vi "Substract Background.vi"(4 "Background":T1, 5 "Substract":u16(ring) items=["None", "Background", "Reference"], 6 "error in (no error)":errorcluster, 7 "Reference":T1, 8 "Dest Img":T1, 9 "Region of Interest":i32[](array[numeric])=[-1, -1, 32000, 32000], 10 "Image Src":T1) -> (0 "error out":errorcluster, 3 "Img Out":T1)   [LabVIEW 2013]
uses:
  <vilib>/vision/Image Controls.llb/IMAQ Image.ctl
  <vilib>/vision/NI_Vision_Development_Module.lvlib
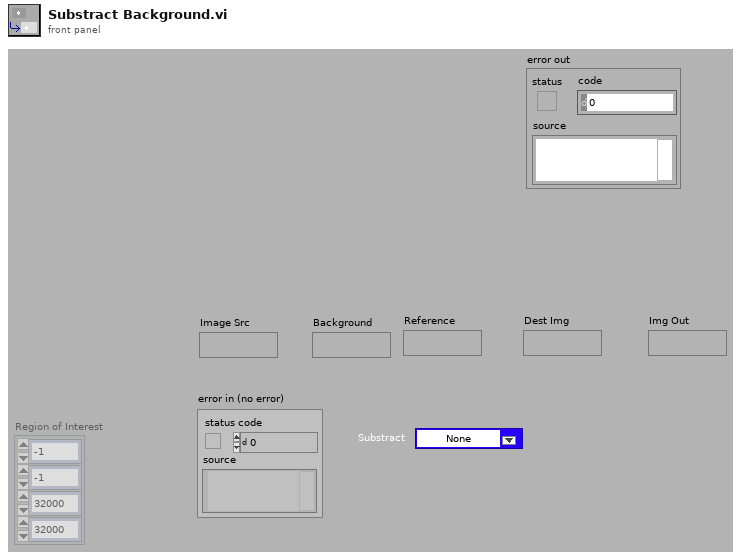
[diagram p1: front panel]
types:
  T1 = typedef "IMAQ Image.ctl" = refnum<image>
  T2 = typedef "Image Type" = u32
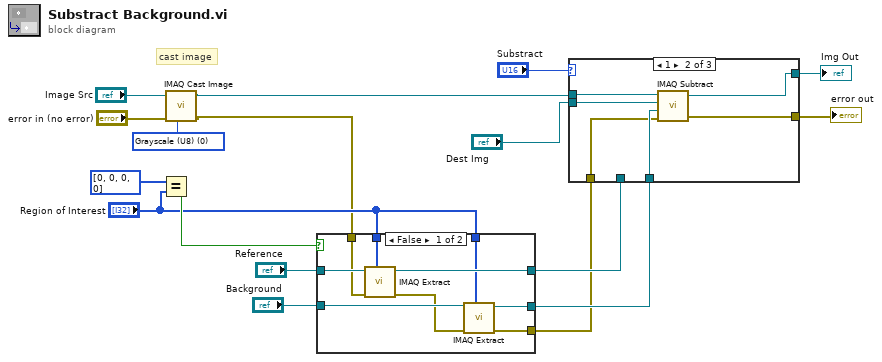
[diagram p0: block diagram]
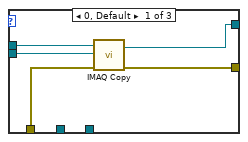
[diagram p3: hidden frame]
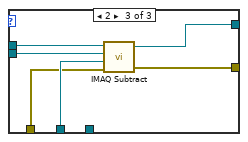
[diagram p4: hidden frame]
diagram:
  w17 = T2 0 items=["Grayscale (U8)", "Grayscale (I16)", "Grayscale (SGL)", "Complex (CSG)", "RGB (U32)", "HSL (U32)", "RGB (U64)", "Grayscale (U16)"] ("Image Type")
  # "cast image"
  n1 = Equal?(x=i32[] [0, 0, 0, 0] ("Region of Interest"), y="Region of Interest") -> (x = y?=w5:bool)
  n2 = call "IMAQ Cast Image"("Image Type"=w17, "error in (no error)"="error in (no error)", "Image Src"="Image Src") -> ("error out"=w1:errorcluster, "Image Dst Out"=w2:T1)  [unwired: 3 in, 4 out]
  n3 = case shown="False" w5 {
    tunnel: "Reference" -> [w26 w29]
    tunnel: "Background" -> [w25 w28]
    tunnel: [w23 w29] -> w6
    tunnel: [w22 w28] -> w7
    tunnel: w1 -> [w21 w27]
    tunnel: "Region of Interest" -> [w20 _]
    tunnel: "Region of Interest" -> [w19 _]
    tunnel: [w18 w27] -> w3
    frame False {
      n4 = call "IMAQ Extract"("Optional Rectangle"=w20, "error in (no error)"=w21, "Image Src"=w26) -> ("error out"=w24:errorcluster, "Image Dst Out"=w23:T1)  [unwired: 7 in]
      n5 = call "IMAQ Extract"("Optional Rectangle"=w19, "error in (no error)"=w24, "Image Src"=w25) -> ("error out"=w18:errorcluster, "Image Dst Out"=w22:T1)  [unwired: 7 in]
    }
    frame True {
    }
  }
  n6 = case shown="1" "Substract" {
    tunnel: w2 -> [w34 w36 w46]
    tunnel: [w30 w40 w45] -> w13
    tunnel: "Dest Img" -> [w33 w35 w44]
    tunnel: [w32 w39 w43] -> w11
    tunnel: w7 -> [_ w38 _]
    tunnel: w6 -> [_ _ w42]
    tunnel: w3 -> [w31 w37 w41]
    frame 0, Default {
      n7 = call "IMAQ Copy"("error in (no error)"=w31, "Image Dst"=w33, "Image Src"=w34) -> ("error out"=w30:errorcluster, "Image Dst Out"=w32:T1)  [unwired: 3 in]
    }
    frame 1 {
      n8 = call "IMAQ Subtract"("Image Src A"=w36, "Image Dst"=w35, "Image Src B"=w38, "error in (no error)"=w37) -> ("Image Dst Out"=w39:T1, "error out"=w40:errorcluster)  [unwired: 3 in]
    }
    frame 2 {
      n9 = call "IMAQ Subtract"("Image Src A"=w46, "Image Dst"=w44, "Image Src B"=w42, "error in (no error)"=w41) -> ("Image Dst Out"=w43:T1, "error out"=w45:errorcluster)  [unwired: 3 in]
    }
  }
  "error out" <- w13
  "Img Out" <- w11
